vi "kanaly array to kanal ctl.vi"(11 "Chan":i32) -> (3 "Kanal":T1)   [LabVIEW 2014]
uses:
  Kontrolki/GUI/RejWol_numer_kanalu.ctl
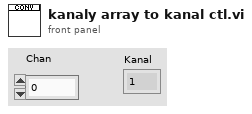
[diagram p1: front panel]
types:
  T1 = typedef "RejWol_numer_kanalu.ctl" = enum16{"1", "2", "3", "4", "5", "6", "7", "8"}
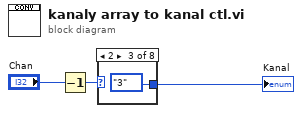
[diagram p0: block diagram]
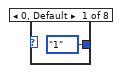
[diagram p2: hidden frame]
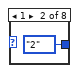
[diagram p3: hidden frame]
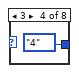
[diagram p4: hidden frame]
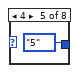
[diagram p5: hidden frame]
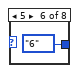
[diagram p6: hidden frame]
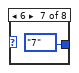
[diagram p7: hidden frame]
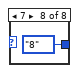
[diagram p8: hidden frame]
diagram:
  n1 = Decrement(x="Chan") -> (x-1=w1:i32)
  n2 = case shown="2" w1 {
    tunnel: [RejWol_numer_kanalu."1" ("Kana³ 1") RejWol_numer_kanalu."2" ("Kana³ 1") RejWol_numer_kanalu."3" ("Kana³ 1") RejWol_numer_kanalu."4" ("Kana³ 1") RejWol_numer_kanalu."5" ("Kana³ 1") RejWol_numer_kanalu."6" ("Kana³ 1") RejWol_numer_kanalu."7" ("Kana³ 1") RejWol_numer_kanalu."8" ("Kana³ 1")] -> w3
    frame 0, Default {
    }
    frame 1 {
    }
    frame 2 {
    }
    frame 3 {
    }
    frame 4 {
    }
    frame 5 {
    }
    frame 6 {
    }
    frame 7 {
    }
  }
  "Kanal" <- w3
